vi "Test-client-limit.vi"(8 "error in (no error)":errorcluster, 10 "Module type":T1, 11 "ModComm in":T2) -> (0 "error out":errorcluster, 1 "Client allowed?":bool, 2 "Module type dup":T1, 3 "ModComm out":T2)   [LabVIEW 2013, in "Server.lvlib" / "Server.lvclass"]
uses:
  Server.lvclass
  Object-reference.ctl
  Supported-module-types.ctl
  UI-messages.ctl
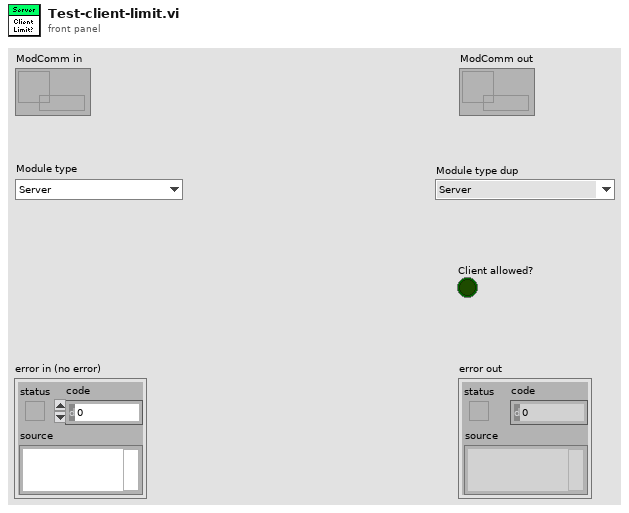
[diagram p1: front panel]
types:
  T1 = typedef "Server.lvlib/Server.lvclass/Supported-module-types.ctl" = enum16{"Server", "All", "BeamControl", "PowderDeposition", "StrategyParser", "CameraVision", "MaterialCharacterization", "StatusMonitor", "SLMSimulation", "LaserCharacterization"}
  T2 = typedef "Server.lvlib/Server.lvclass/Object-reference.ctl" = refnum<data-value>
  T3 = typedef "Server.lvlib/Server.lvclass/UI-messages.ctl" = enum16{"Time out", "User cancel", "Module cancel", "Client inactivity", "Client limit", "Client started"}
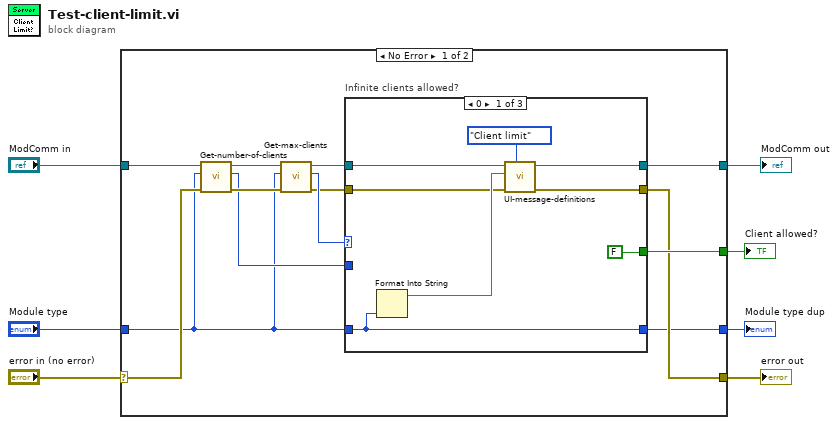
[diagram p0: block diagram]
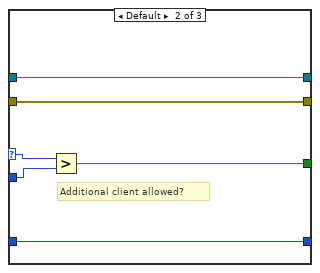
[diagram p2: hidden frame]
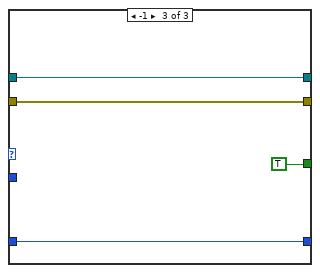
[diagram p3: hidden frame]
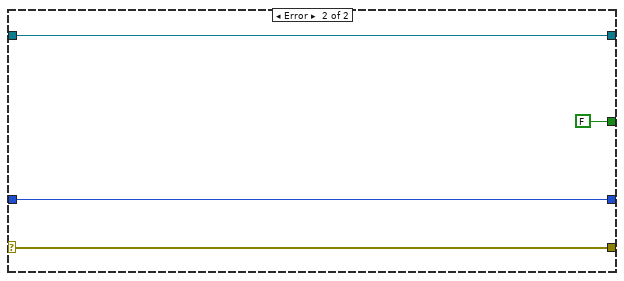
[diagram p4: hidden frame]
diagram:
  n1 = case shown="No Error" "error in (no error)" {
    selector: "error in (no error)" -> [w15 w42]
    tunnel: [w9 w42] -> w6
    tunnel: [w10 w41] -> w4
    tunnel: "ModComm in" -> [w20 w41]
    tunnel: "Module type" -> [w11 w39]
    tunnel: [w14 FALSE] -> w2
    tunnel: [w8 w39] -> w1
    frame No Error {
      n2 = call "Get-number-of-clients.vi"("error in (no error)"=w15, "Module type"=w11, "ModComm in"=w20) -> ("error out"=w18:errorcluster, "# clients"=w16:i32, "ModComm out"=w19:T2)  [unwired: 6 in]
      n3 = call "Get-max-clients.vi"("error in (no error)"=w18, "Module type"=w11, "ModComm in"=w19) -> ("error out"=w12:errorcluster, "Max clients"=w17:i32, "ModComm out"=w13:T2)  [unwired: 6 in]
      n4 = case "Infinite clients allowed?" shown="0" w17 {
        selector: w17 -> [_ w34 _]
        tunnel: w16 -> [_ w33 _]
        tunnel: [FALSE w32 TRUE] -> w14
        tunnel: w13 -> [w26 w31 w37]
        tunnel: w12 -> [w24 w30 w36]
        tunnel: w11 -> [w21 w29 w35]
        tunnel: [w23 w31 w37] -> w10
        tunnel: [w22 w30 w36] -> w9
        tunnel: [w21 w29 w35] -> w8
        frame 0 {
          n5 = Format Into String(w21) -> (resulting string=w25:string)  [unwired: 3 in, 1 out]
          n6 = call "UI-message-definitions.vi"("Message"=UI-messages."Client limit", "error in (no error)"=w24, "Additional text"=w25, "ModComm in"=w26) -> ("error out"=w22:errorcluster, "ModComm out"=w23:T2)  [unwired: 6 in]
        }
        frame Default {
          # "Additional client allowed?"
          n7 = Greater?(x=w34, y=w33) -> (0:w32:bool)
        }
        frame -1 {
        }
      }
    }
    frame Error {
    }
  }
  "error out" <- w6
  "ModComm out" <- w4
  "Client allowed?" <- w2
  "Module type dup" <- w1
